vi "FPGA Global.vi"() -> ()   [LabVIEW 2011]
panel:
  out "Control Inputs Valid":bool
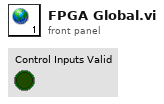
[diagram p1: front panel]
diagram:
